vi "SW_Check_password.vi"(8 "error in (no error)":errorcluster, 9 "Entered key":T3, 10 "Controls references":T1, 11 "Configuration file refnum in":T2) -> (0 "error out":errorcluster, 3 "Stop the loop":bool)   [LabVIEW 2016]
uses:
  <vilib>/event_ctls.llb/eventvkey.ctl
  <vilib>/Utility/config.llb/Config Data RefNum.ctl
  <vilib>/Utility/config.llb/NI_LVConfig.lvlib
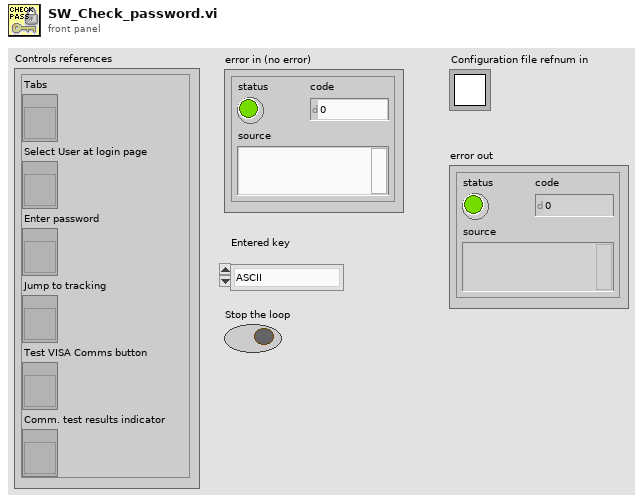
[diagram p1: front panel]
types:
  T1 = cluster{"Tabs":refnum<vi>, "Select User at login page":refnum<vi>, "Enter password":refnum<vi>, "Jump to tracking":refnum<vi>, "Test VISA Comms button":refnum<vi>, "Comm. test results indicator":refnum<vi>}
  T2 = typedef "NI_LVConfig.lvlib/Config Data RefNum.ctl" = refnum<k1>
  T3 = typedef "eventvkey.ctl" = enum16{"ASCII", "Enter", "Return", "Shift", "Ctrl", "Alt", "Cmd", "Opt", "Caps", "NumLock", "Clear", "Break", "Up", "Down", "Left", "Right", "Insert", "Delete", "Home", "End", "PageUp", "PageDown", "Escape", "Help", "Pause", "ScrollLock", "F1", "F2", "F3", "F4", "F5", "F6", "F7", "F8", "F9", "F10", "F11", "F12", "F13", "F14", "F15", "F16", "F17", "F18", "F19", "F20", "F21", "F22", "F23", "F24", "Play", "VolumeUp", "VolumeDown", "Mute", "Two Byte Char"}
  T4 = enum8{"Enabled", "Disabled", "Disabled and Grayed Out"}
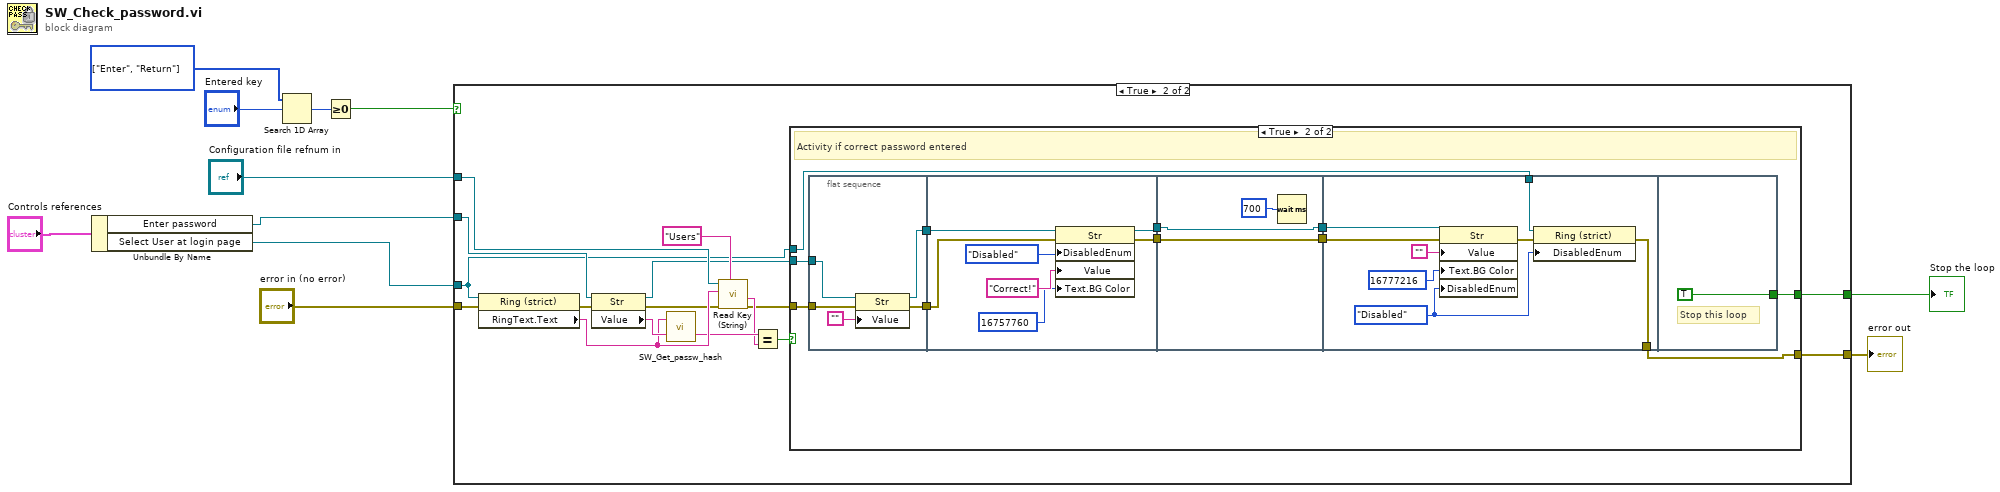
[diagram p0: block diagram]
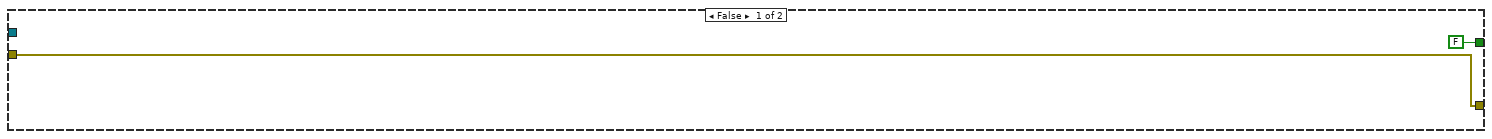
[diagram p2: hidden frame]
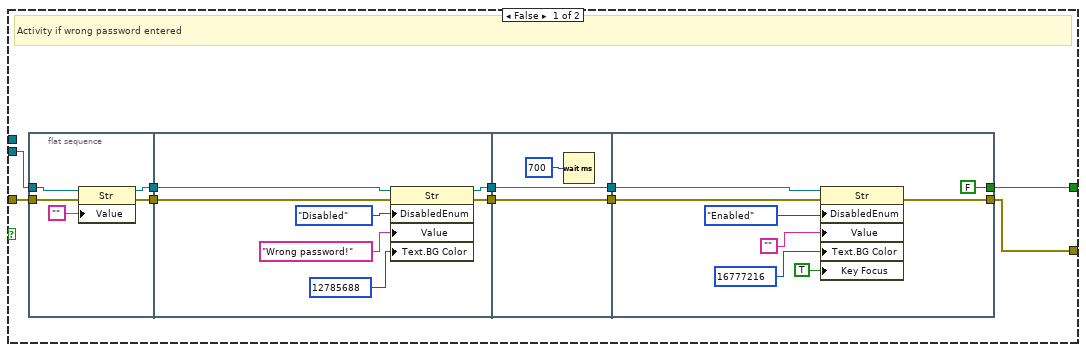
[diagram p3: hidden frame]
diagram:
  w7 = T3[] [enum."Enter", enum."Return"] items=["ASCII", "Enter", "Return", "Shift", "Ctrl", "Alt", "Cmd", "Opt", "Caps", "NumLock", "Clear", "Break", "Up", "Down", "Left", "Right", "Insert", "Delete", "Home", "End", "PageUp", "PageDown", "Escape", "Help", "Pause", "ScrollLock", "F1", "F2", "F3", "F4", "F5", "F6", "F7", "F8", "F9", "F10", "F11", "F12", "F13", "F14", "F15", "F16", "F17", "F18", "F19", "F20", "F21", "F22", "F23", "F24", "Play", "VolumeUp", "VolumeDown", "Mute", "Two Byte Char"] ("1D array")
  n1 = Unbundle By Name("Controls references") -> ("Enter password"=w1:refnum<vi>, "Select User at login page"=w2:refnum<vi>)
  n2 = Search 1D Array(1D array=w7, element="Entered key") -> (index of element=w9:i32)  [unwired: 1 in]
  n3 = Greater Or Equal To 0?(x=w9) -> (x >= 0?=w8:bool)
  n4 = case shown="True" w8 {
    tunnel: "Configuration file refnum in" -> [_ w27]
    tunnel: [FALSE w20] -> w10
    tunnel: [w12 w19] -> w11
    tunnel: w2 -> [_ w15]
    tunnel: w1 -> [_ w16]
    tunnel: "error in (no error)" -> [w12 w14]
    frame False {
    }
    frame True {
      n5 = property on="Property Node" class="Ring (strict)"(reference=w15, error in=w14) -> (error out=w28:errorcluster, "RingText.Text"=w26:string)  [unwired: 1 out]
      n6 = property on="Property Node" class="Str"(reference=w16, error in=w28) -> (reference out=w17:refnum<vi>, error out=w25:errorcluster, "Value"=w29:string)
      n7 = call "SW_Get_passw_hash.vi"("Password"=w29, "Username"=w26) -> ("Password hash"=w24:string)  [unwired: 1 out]
      n8 = call <vilib>:"Read Key (String).vi"("section"="Users", "error in (no error)"=w25, "key"=w26, "refnum"=w27) -> ("error out"=w21:errorcluster, "value"=w23:string)  [unwired: 4 in, 2 out]
      n9 = Equal?(x=w24, y=w23) -> (x = y?=w22:bool)
      n10 = case shown="True" w22 {
        tunnel: w21 -> [w39 w70]
        tunnel: [w35 w69] -> w20
        tunnel: [w34 w68] -> w19
        tunnel: w17 -> [w33 w67]
        tunnel: w15 -> [_ w66]
        frame False {
          # "Activity if wrong password entered"
          n11 = flat-sequence {
            tunnel: w39 -> [w43]
            tunnel: [w42] -> w38
            tunnel: w33 -> [w41]
            tunnel: [w40] -> w32
            tunnel: w38 -> [w49]
            tunnel: [w48] -> w36
            tunnel: w32 -> [w46]
            tunnel: [w45] -> w30
            tunnel: [w53] -> w37
            tunnel: w36 -> [w53]
            tunnel: [w52] -> w31
            tunnel: w30 -> [w52]
            tunnel: w37 -> [w60]
            tunnel: [FALSE] -> w35
            tunnel: [w56] -> w34
            tunnel: w31 -> [w55]
            frame #0 {
              n12 = property on="Property Node" class="Str"(reference=w41, error in=w43, "Value"="") -> (reference out=w40:refnum<vi>, error out=w42:errorcluster)
            }
            frame #1 {
              n13 = property on="Property Node" class="Str"(reference=w46, error in=w49, "DisabledEnum"=T4."Disabled" ("Disabled"), "Value"="Wrong password!" ("Enter password"), "Text.BG Color"=u32 12785688 ("Text.Colors:BG Color")) -> (reference out=w45:refnum<vi>, error out=w48:errorcluster)
            }
            frame #2 {
              n14 = Wait (ms)(milliseconds to wait=u32 700) -> ()  [unwired: 1 out]
            }
            frame #3 {
              n15 = property on="Property Node" class="Str"(reference=w55, error in=w60, "DisabledEnum"=T4."Enabled" ("Disabled"), "Value"="", "Text.BG Color"=u32 16777216 ("Text.Colors:BG Color"), "Key Focus"=TRUE) -> (error out=w56:errorcluster)  [unwired: 1 out]
            }
          }
        }
        frame True {
          # "Activity if correct password entered"
          n16 = flat-sequence {
            tunnel: w70 -> [w77]
            tunnel: [w76] -> w73
            tunnel: w67 -> [w75]
            tunnel: [w74] -> w65
            tunnel: w73 -> [w83]
            tunnel: [w82] -> w72
            tunnel: w65 -> [w80]
            tunnel: [w79] -> w63
            tunnel: [w87] -> w71
            tunnel: w72 -> [w87]
            tunnel: [w86] -> w64
            tunnel: w63 -> [w86]
            tunnel: w71 -> [w95]
            tunnel: [w91] -> w68
            tunnel: w66 -> [w90]
            tunnel: w64 -> [w89]
            tunnel: [TRUE] -> w69
            frame #0 {
              n17 = property on="Property Node" class="Str"(reference=w75, error in=w77, "Value"="") -> (reference out=w74:refnum<vi>, error out=w76:errorcluster)
            }
            frame #1 {
              n18 = property on="Property Node" class="Str"(reference=w80, error in=w83, "DisabledEnum"=T4."Disabled" ("Disabled"), "Value"="Correct!" ("Enter password"), "Text.BG Color"=u32 16757760 ("Text.Colors:BG Color")) -> (reference out=w79:refnum<vi>, error out=w82:errorcluster)
            }
            frame #2 {
              n19 = Wait (ms)(milliseconds to wait=u32 700) -> ()  [unwired: 1 out]
            }
            frame #3 {
              w93 = T4."Disabled" ("Disabled")
              n20 = property on="Property Node" class="Str"(reference=w89, error in=w95, "Value"="", "Text.BG Color"=u32 16777216 ("Text.Colors:BG Color"), "DisabledEnum"=w93) -> (error out=w92:errorcluster)  [unwired: 1 out]
              n21 = property on="Property Node" class="Ring (strict)"(reference=w90, error in=w92, "DisabledEnum"=w93) -> (error out=w91:errorcluster)  [unwired: 1 out]
            }
            frame #4 {
              # "Stop this loop"
            }
          }
        }
      }
    }
  }
  "error out" <- w11
  "Stop the loop" <- w10
